vi "1DFloat64ArrayToNode(viaString).vi"(0 "Tree DVR in":refnum<data-value>, 1 "DBL Array":dbl[](array[numeric]), 3 "error in (no error)":errorcluster, 4 "NodePath":string) -> (5 "Tree DVR out":refnum<data-value>, 7 "error out":errorcluster)   [LabVIEW 2014]
uses:
  <vilib>/MDSplus/Classes/Tree_Class/Tree.lvclass
  <vilib>/MDSplus/Library/MDSplus.lvlib
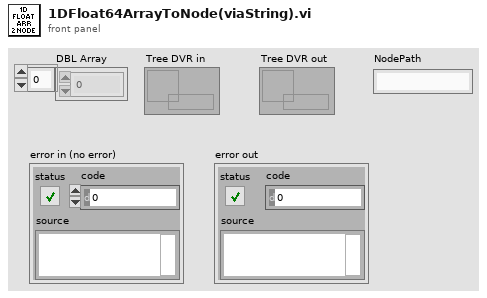
[diagram p1: front panel]
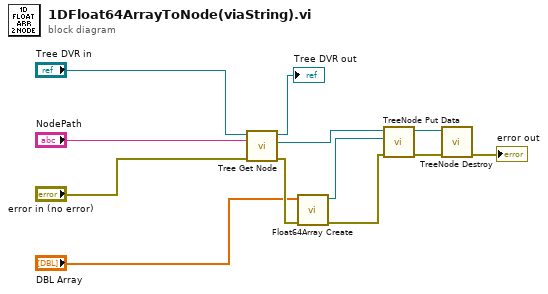
[diagram p0: block diagram]
diagram:
  n1 = call <vilib>:"Tree Get Node.vi"("error in (no error)"="error in (no error)", "Path"="NodePath", "Tree DVR in"="Tree DVR in") -> ("error out"=w8:errorcluster, "Node out"=w5:refnum<data-value>, "Tree DVR out"=→"Tree DVR out":refnum<data-value>)  [unwired: 6 in]
  n2 = call <vilib>:"Float64Array Create.vi"("error in (no error)"=w8, "DBL array in"="DBL Array") -> ("error out"=w7:errorcluster, "Float64Array DVR out"=w4:refnum<data-value>)  [unwired: 8 in]
  n3 = call <vilib>:"TreeNode Put Data.vi"("error in (no error)"=w7, "Data"=w4, "TreeNode DVR in"=w5) -> ("error out"=w2:errorcluster, "TreeNode DVR out"=w1:refnum<data-value>)  [unwired: 7 in]
  n4 = call <vilib>:"TreeNode Destroy.vi"("error in (no error)"=w2, "TreeNode DVR in"=w1) -> ("error out"=→"error out":errorcluster)  [unwired: 9 in]
